vi "Calculate index v0.3.vi"(3 "Central Wavelength":dbl=600.0 format="%.2f", 4 "Current Wavelength":dbl=600.0 format="%.2f", 5 "Current Grating Density":enum16{"150", "300", "600", "1200", "1800"}(ring)=enum."600" caption="Grating Density") -> (1 "index (out)":dbl=571.2504622529284 format="%.4f")   [LabVIEW 2019]
panel:
  out "Detector Pixel Distance":dbl=27.0 format="%.2f"
  out "Spectrometer Mirror angle":dbl=21.18 format="%.2f"
  out "Spectrometer Focal length":dbl=750.0 format="%.1f"
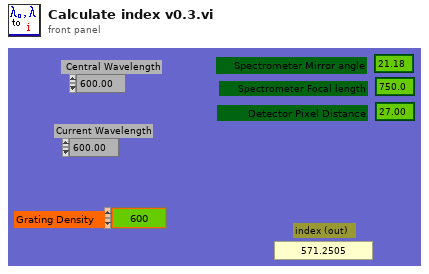
[diagram p1: front panel]
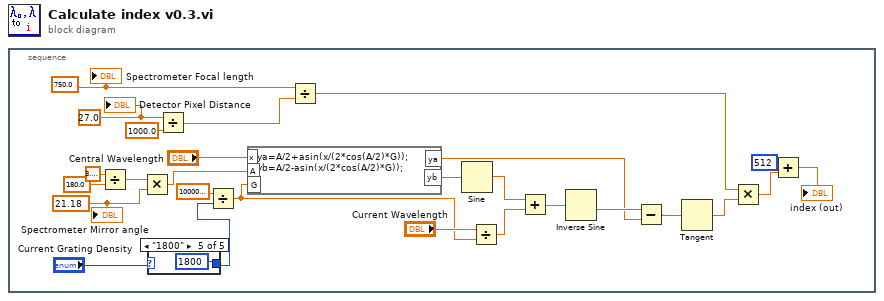
[diagram p0: block diagram]
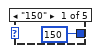
[diagram p2: hidden frame]
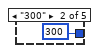
[diagram p3: hidden frame]
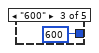
[diagram p4: hidden frame]
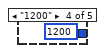
[diagram p5: hidden frame]
diagram:
  n1 = stacked-sequence {
    frame #0 {
      w23 = 21.18 ("Detector Pixel Distance")
      w16 = 750.0 ("Detector Pixel Distance")
      w24 = 27.0 ("x")
      n2 = Divide(x=3.141592653589793, y=180.0) -> (x/y=w21:dbl)
      n3 = Multiply(x=w21, y=w23) -> (x*y=w22:dbl)
      n4 = case shown="\"1800\"" "Current Grating Density" {
        tunnel: [150 300 600 1200 1800] -> w18
        frame "150" {
        }
        frame "300" {
        }
        frame "600" {
        }
        frame "1200" {
        }
        frame "1800" {
        }
      }
      n5 = Divide(x=w24, y=1000.0) -> (x/y=w15:dbl)
      n6 = Divide(x=1000000.0, y=w18) -> (x/y=w12:dbl)
      n7 = formula code="ya=A/2+asin(x/(2*cos(A/2)*G));\nyb=A/2-asin(x/(2*cos(A/2)*G));"("x"="Central Wavelength", "A"=w22, "G"=w12) -> ("ya"=w7:dbl, "yb"=w13:dbl)
      n8 = Divide(x=w16, y=w15) -> (x/y=w4:dbl)
      n9 = Sine(x=w13) -> (sin(x)=w11:dbl)
      n10 = Divide(x="Current Wavelength", y=w12) -> (x/y=w10:dbl)
      n11 = Add(x=w11, y=w10) -> (x+y=w9:dbl)
      n12 = Inverse Sine(1:w9) -> (0:w8:dbl)
      n13 = Subtract(x=w8, y=w7) -> (x-y=w6:dbl)
      n14 = Tangent(1:w6) -> (0:w5:dbl)
      n15 = Multiply(x=w4, y=w5) -> (x*y=w2:dbl)
      n16 = Add(x=512, y=w2) -> (x+y=→"index (out)":dbl)
      "Spectrometer Focal length" <- w16
      "Spectrometer Mirror angle" <- w23
      "Detector Pixel Distance" <- w24
    }
  }
